vi "AppendOrReplace.vi"(9 "index 2":i32, 10 "new element/subarray 2":dbl[][](array[numeric]), 11 "Sequence 2":dbl[][][](array[numeric])) -> (3 "Sequence":dbl[][][](array[numeric]))   [LabVIEW 2017, in "AODControl.lvlib"]
uses:
  AODControl.lvlib
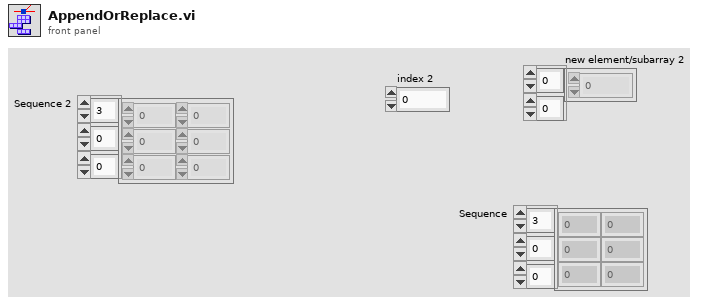
[diagram p1: front panel]
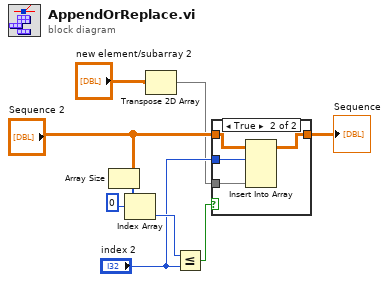
[diagram p0: block diagram]
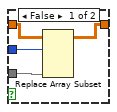
[diagram p2: hidden frame]
diagram:
  n1 = Array Size(array="Sequence 2") -> (size(s)=w8:i32[])
  n2 = Index Array(array=w8, index=0) -> (element=w6:i32)
  n3 = Transpose 2D Array(2D array="new element/subarray 2") -> (transposed array=w1:dbl[][])
  n4 = Less Or Equal?(x=w6, y="index 2") -> (x <= y?=w5:bool)
  n5 = case shown="True" w5 {
    tunnel: [w13 w16] -> w7
    tunnel: "Sequence 2" -> [w12 w17]
    tunnel: w1 -> [w11 w14]
    tunnel: "index 2" -> [w10 w15]
    frame False {
      n6 = Replace Array Subset(array=w12, new element=w11, index (dim 0)=w10) -> (w13:dbl[][][])  [unwired: 2 in]
    }
    frame True {
      n7 = Insert Into Array(array=w17, index (dim 0)=w15, new element=w14) -> (w16:dbl[][][])  [unwired: 2 in]
    }
  }
  "Sequence" <- w7
